vi "Unique Numbers and Multiplicity.vi"   [LabVIEW 2010, in "NI_AALPro.lvlib"]
doc: "Obtains all the unique numbers from the input array and determines the multiplicity of each unique number. Wire data to the <B>Numbers</B> input to determine the polymorphic instance to use or manually select the instance."
uses:
  NI_AALPro.lvlib
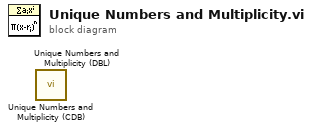
[diagram p0: block diagram]
diagram:
  n1 = call "Unique Numbers and Multiplicity (CDB).vi"() -> ()  [unwired: 9 in, 3 out]
  n2 = call "Unique Numbers and Multiplicity (DBL).vi"() -> ()  [unwired: 9 in, 3 out]
